vi "q1 previous current value feedback.vi"() -> ()   [LabVIEW 2025]
panel:
  in  "stop":bool
  out "previous":dbl
  out "current":dbl
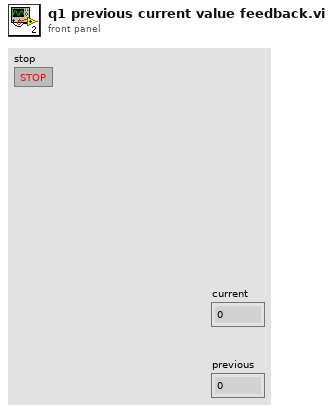
[diagram p1: front panel]
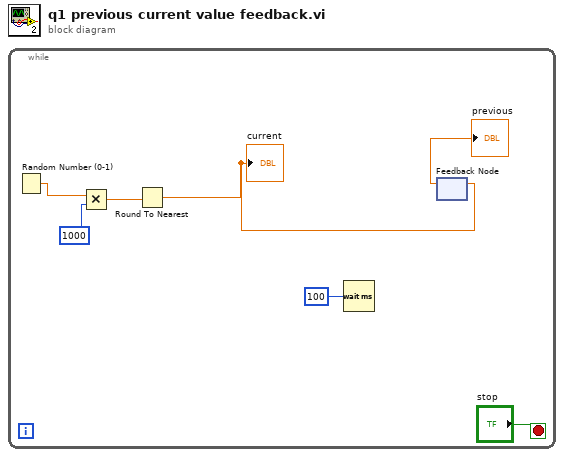
[diagram p0: block diagram]
diagram:
  n1 = while {
    stop <- "stop" stop-if-true
    n2 = Random Number (0-1)() -> (number: 0 to 1=w4:dbl)
    n3 = Multiply(x=w4, y=1000) -> (x*y=w2:dbl)
    n4 = Round To Nearest(number=w2) -> (nearest integer value=w1:dbl)
    "current" <- w1
    n5 = Wait (ms)(milliseconds to wait=100) -> ()  [unwired: 1 out]
    n6 = feedback-in #1(w1) -> ()
    n7 = feedback #1() -> (→"previous":dbl)  [unwired: 1 in]
  }
